vi "NIDCPower_channel_ganging - initialize.vi"(6 "Ganged Config":T2, 7 "option string":string="Simulate=0", 8 "error in (no error)":errorcluster, 9 "reset (false)":bool, 11 "Channel List":T4[](array[typedef])) -> (0 "error out":errorcluster, 3 "Ganged Session Out":T1)   [LabVIEW 2021]
doc: "Creates a new NI-DCPower_channel_ganging session to the specified instrument(s) and channel(s) and returns a session handle to be used in all subsequent NI-DCPower_channel_ganging VI calls.\n\nAfter calling this VI, the specified channel or channels will be in the Uncommitted state."
uses:
  ctl/NIDCPower_channel_ganging - ctl - channel def.ctl
  ctl/NIDCPower_channel_ganging - ctl - channel mode.ctl
  ctl/NIDCPower_channel_ganging - ctl - ganged config.ctl
  ctl/NIDCPower_channel_ganging - ctl - ganged session.ctl
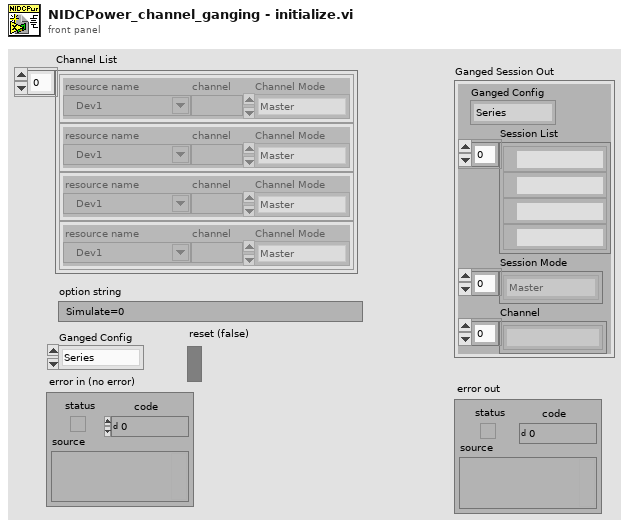
[diagram p1: front panel]
types:
  T1 = typedef "NIDCPower_channel_ganging - ctl - ganged session.ctl" = cluster{"Ganged Config":T2, "Session List":refnum<k15>[], "Session Mode":T3[], "Channel":string[]}
  T2 = typedef "NIDCPower_channel_ganging - ctl - ganged config.ctl" = enum32{"Series", "Parallel", "Manual"}
  T3 = typedef "NIDCPower_channel_ganging - ctl - channel mode.ctl" = enum32{"Master", "Slave", "Slave - Inverted"}
  T4 = typedef "NIDCPower_channel_ganging - ctl - channel def.ctl" = cluster{"resource name":refnum<k15>, "channels":string, "Channel Mode":T3}
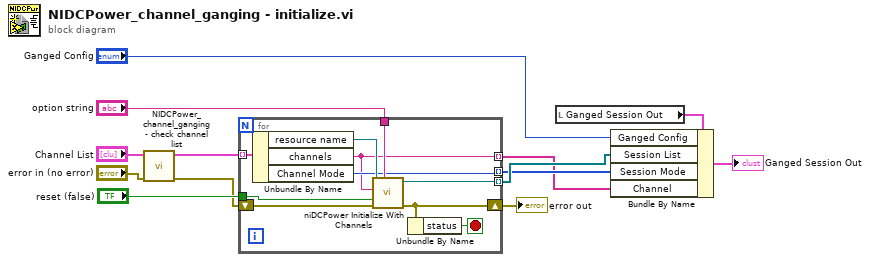
[diagram p0: block diagram]
diagram:
  n1 = call "NIDCPower_channel_ganging - check channel list.vi"("error in (no error)"="error in (no error)", "Channel List In"="Channel List") -> ("error out"=w7:errorcluster, "Channel List Out"=w10:T4[])  [unwired: 8 in]
  n2 = for {
    shift-right: [w17] -> w13
    shift-left: w7 -> [w23]
    tunnel: w10 -> [w22] mode=indexing
    tunnel: "reset (false)" -> [w20]
    tunnel: "option string" -> [w19]
    tunnel: [w18] -> w5 mode=indexing
    tunnel: [w15] -> w2 mode=indexing
    tunnel: [w14] -> w1 mode=indexing
    stop <- w16 stop-if-true
    n3 = Unbundle By Name(w22) -> ("resource name"=w21:refnum<k15>, "channels"=w14:string, "Channel Mode"=w15:T3)
    n4 = call <instrlib>:"niDCPower Initialize With Channels.vi"("option string"=w19, "error in (no error)"=w23, "reset (false)"=w20, "channels"=w14, "resource name"=w21) -> ("error out"=w17:errorcluster, "instrument handle out"=w18:refnum<k15>)  [unwired: 5 in]
    n5 = Unbundle By Name(w17) -> ("status"=w16:bool)
  }
  "error out" <- w13
  n6 = local read "Ganged Session Out"() -> (w3:T1)
  n7 = Bundle By Name(cluster=w3, "Ganged Config"="Ganged Config", "Session List"=w5, "Session Mode"=w2, "Channel"=w1) -> (→"Ganged Session Out":T1)
